vi "brc_daq_connect_module.vi"(11 "index":i32) -> (0 "error out":errorcluster, 3 "return_value":i32)   [LabVIEW 2015, in "BRC-DAQ x86.lvlib"]
uses:
  BRC-DAQ x86.lvlib
  DLL/brc_daq_sdk.dll
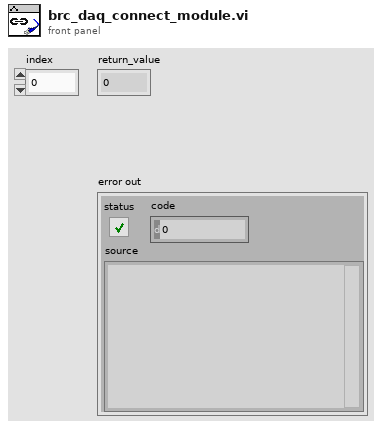
[diagram p1: front panel]
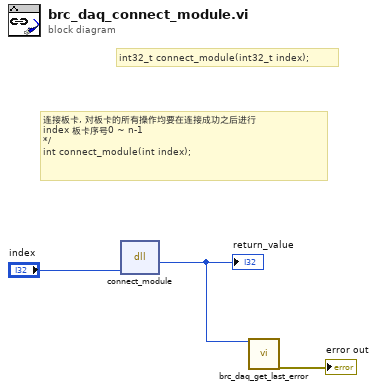
[diagram p0: block diagram]
diagram:
  # "int32_t connect_module(int32_t index);"
  # "连接板卡, 对板卡的所有操作均要在连接成功之后进行\nindex 板卡序号0 ~ n-1\n*/\nint connect_module(int index);"
  n1 = dll-call lib="E:/01 BRC project/04BRC-daq/04 Drive/BRC-DAQ/DAQ-x86/DLL/brc_daq_sdk.dll" fn="connect_module"("index"="index") -> ("return type"=w2:i32)  [unwired: 4 in, 2 out]
  "return_value" <- w2
  n2 = call "brc_daq_get_last_error.vi"("return_value"=w2) -> ("error out"=→"error out":errorcluster)  [unwired: 18 in]
